vi "ColorAbsort.vi"(8 "error in (no error)":errorcluster caption="错误输入（无错误）", 9 "位置":cluster{"X":i32, "Y":i32}, 10 "图片宽":i16, 11 "image":u8[](array[numeric])) -> (0 "error out":errorcluster caption="错误输出", 1 "B":u8, 2 "G":u8, 3 "R":u8, 4 "颜色盒":u32(colorbox))   [LabVIEW 2015]
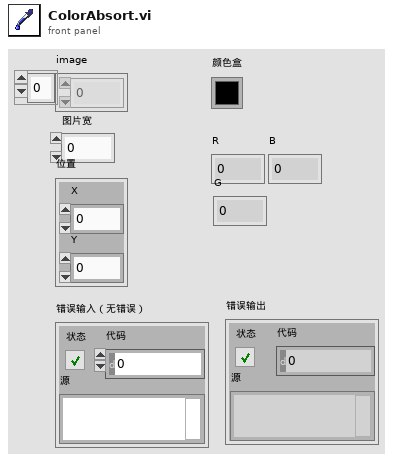
[diagram p1: front panel]
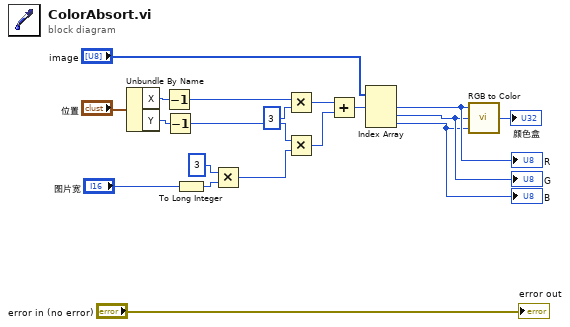
[diagram p0: block diagram]
diagram:
  n1 = Unbundle By Name("位置") -> ("X"=w12:i32, "Y"=w11:i32)
  n2 = Decrement(x=w12) -> (x-1=w9:i32)
  n3 = Decrement(x=w11) -> (x-1=w10:i32)
  n4 = To Long Integer(number="图片宽") -> (32bit integer=w7:i32)
  n5 = Multiply(x=3, y=w7) -> (x*y=w4:i32)
  n6 = Multiply(x=w9, y=3) -> (x*y=w17:i32)
  n7 = Multiply(x=w10, y=w4) -> (x*y=w18:i32)
  n8 = Add(x=w17, y=w18) -> (x+y=w19:i32)
  n9 = Index Array(array="image", index #1=w19) -> (element #1=w3:u8, element #2=w2:u8, element #3=w1:u8)  [unwired: 2 in]
  "R" <- w3
  "G" <- w2
  "B" <- w1
  n10 = call <vilib>:"RGB to Color.vi"("B"=w1, "G"=w2, "R"=w3) -> ("Color"=→"颜色盒":u32)
  "error out" <- "error in (no error)"
